vi "SendJoystickProtocol.vi"(7 "Send":bool, 9 "Initialize":bool, 10 "Joystick old":T1={"type"="Joystick", "device"="3", "name"="", "data"={"<init"=FALSE, ">buttons"=[], ">povs"=[], ">axes"=[], "<left_rumble"=0.0, "<right_rumble"=0.0, "<outputs"=0}}, 11 "Joystick new":T1={"type"="Joystick", "device"="3", "name"="", "data"={"<init"=FALSE, ">buttons"=[], ">povs"=[], ">axes"=[], "<left_rumble"=0.0, "<right_rumble"=0.0, "<outputs"=0}}) -> ()   [LabVIEW 2019]
uses:
  Joystick proto.ctl
  Joystick data proto.ctl
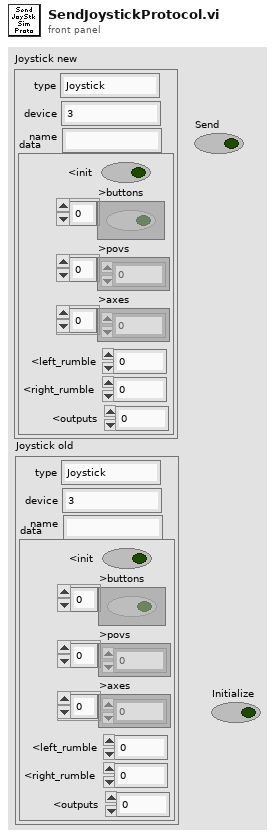
[diagram p1: front panel]
types:
  T1 = typedef "Joystick proto.ctl" = cluster{"type":string, "device":string, "name":string, "data":T2}
  T2 = typedef "Joystick data proto.ctl" = cluster{"<init":bool, ">buttons":bool[], ">povs":i32[], ">axes":i32[], "<left_rumble":dbl, "<right_rumble":dbl, "<outputs":i32}
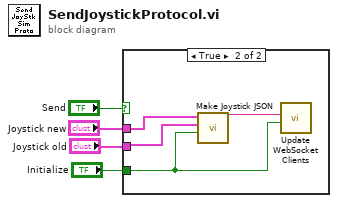
[diagram p0: block diagram]
diagram:
  n1 = case shown="True" "Send" {
    tunnel: "Joystick new" -> [_ w7]
    tunnel: "Joystick old" -> [_ w6]
    tunnel: "Initialize" -> [_ w5]
    frame False {
    }
    frame True {
      n2 = call "Make Joystick JSON.vi"("Force"=w5, "Joystick prev"=w6, "Joystick new"=w7) -> ("JSON delta"=w8:string)  [unwired: 8 in]
      n3 = call "Update WebSocket Clients.vi"("Initialize"=w5, "delta JSON"=w8) -> ()  [unwired: 10 in]
    }
  }
